vi "changeScale.vi"(8 "error in (no error)":errorcluster, 10 "newValue":dbl, 11 "ImageStreamViewer in":refnum<class "ImageStreamViewer.lvclass">) -> (0 "error out":errorcluster, 3 "ImageStreamViewer out":refnum<class "ImageStreamViewer.lvclass">)   [LabVIEW 2011, in "Views.lvlib" / "Camera.lvlib" / "ImageStreamViewer.lvclass"]
uses:
  ImageStreamViewer.lvclass
  ImageStreamViewer.lvclass/ImageStreamViewer.ctl
  <vilib>/vision/NI_Vision_Development_Module.lvlib
panel:
  # "change the image display scale"
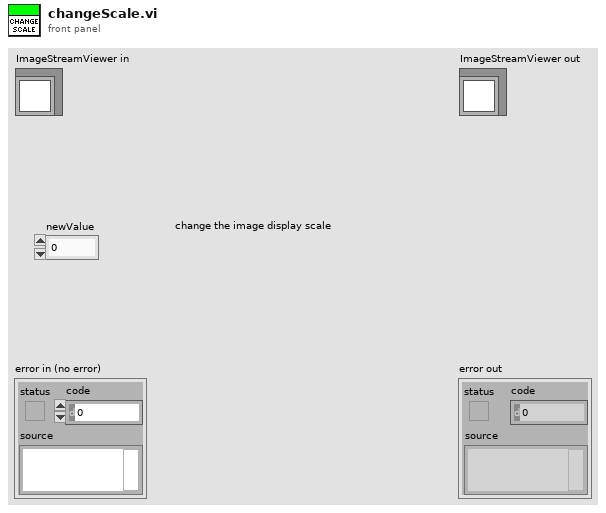
[diagram p1: front panel]
types:
  T1 = typedef "IMAQ Image.ctl" = refnum<image>
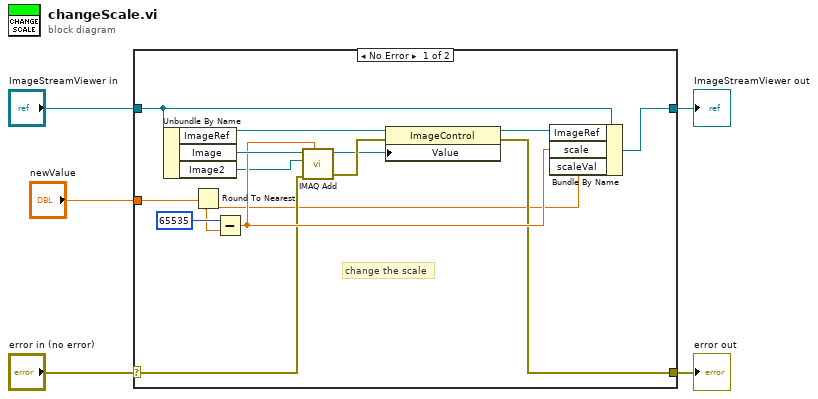
[diagram p0: block diagram]
diagram:
  n1 = case shown="No Error" "error in (no error)" {
    selector: "error in (no error)" -> [w10 w21]
    tunnel: [w9 w21] -> w4
    tunnel: [w7 w20] -> w2
    tunnel: "ImageStreamViewer in" -> [w19 w20]
    tunnel: "newValue" -> [w17 _]
    frame No Error {
      # "change the scale"
      n2 = Unbundle By Name(w19) -> ("ImageRef"=w13:refnum<vi>, "Image"=w16:T1, "Image2"=w14:T1)
      n3 = Round To Nearest(number=w17) -> (nearest integer value=w6:dbl)
      n4 = Subtract(x=65535, y=w6) -> (x-y=w15:dbl)
      n5 = call "IMAQ Add"("Image Src A"=w16, "Constant"=w15, "Image Dst"=w14, "error in (no error)"=w10) -> ("Image Dst Out"=w11:T1, "error out"=w12:errorcluster)  [unwired: 3 in]
      n6 = property class="ImageControl"(reference=w13, error in=w12, "Value"=w11) -> (reference out=w8:refnum<vi>, error out=w9:errorcluster)
      n7 = Bundle By Name(cluster=w19, "ImageRef"=w8, "scale"=w15, "scaleVal"=w6) -> (w7:refnum<class "ImageStreamViewer.lvclass">)
    }
    frame Error {
    }
  }
  "error out" <- w4
  "ImageStreamViewer out" <- w2
